vi "Derivative.vi"(10 "X":dbl[](array[numeric]), 11 "Y":dbl[](array[numeric])) -> (3 "dY/dX":dbl[](array[numeric]))   [LabVIEW 2014]
uses:
  <vilib>/Analysis/NI_AALPro.lvlib
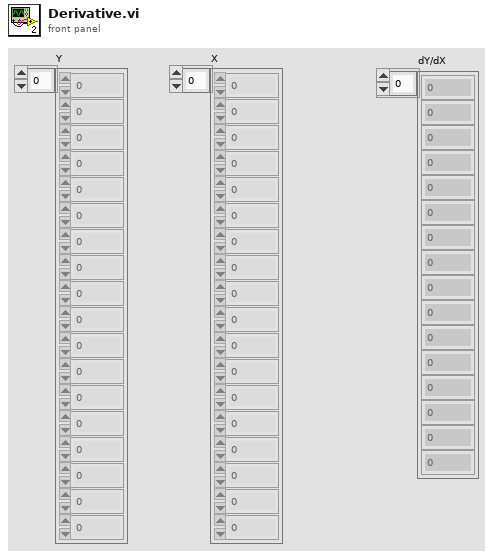
[diagram p1: front panel]
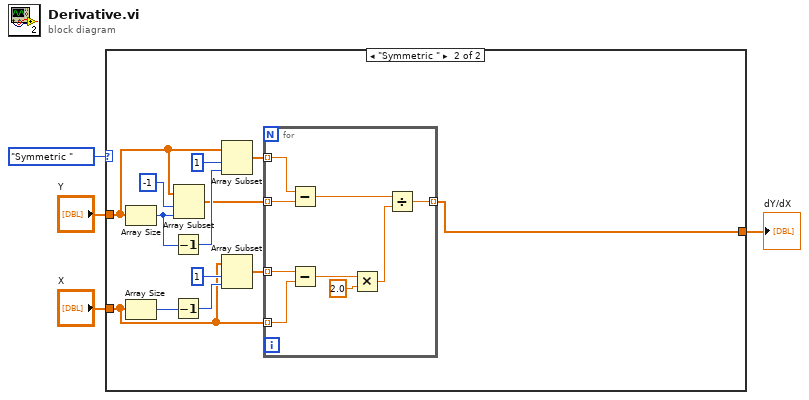
[diagram p0: block diagram]
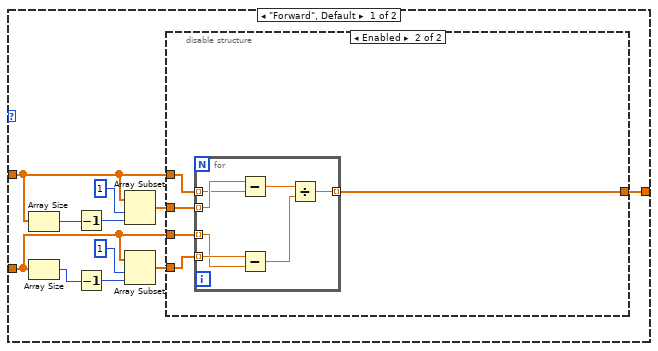
[diagram p2: hidden frame]
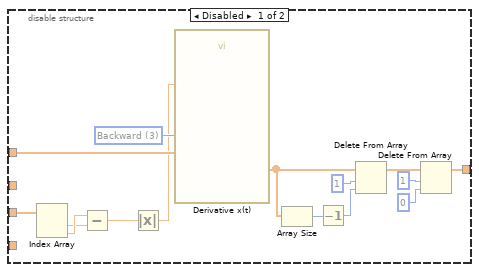
[diagram p3: hidden frame]
diagram:
  n1 = case shown="\"Symmetric \"" enum16{"Forward", "Symmetric "}."Symmetric " {
    tunnel: [w15 w43] -> w4
    tunnel: "Y" -> [w14 w48]
    tunnel: "X" -> [w6 w44]
    frame "Forward", Default {
      n2 = Array Size(array=w14) -> (size(s)=w12:i32)
      n3 = Array Size(array=w6) -> (size(s)=w9:i32)
      n4 = Decrement(x=w12) -> (x-1=w11:i32)
      n5 = Decrement(x=w9) -> (x-1=w8:i32)
      n6 = Array Subset(array=w14, index=1, length=w11) -> (w10:dbl[])
      n7 = Array Subset(array=w6, index=1, length=w8) -> (w5:dbl[])
      n8 = disable-structure shown="Enabled" {
        disable-tunnel: w14 -> [w22 w34]
        disable-tunnel: w6 -> [w21 w35]
        disable-tunnel: [w17 w31] -> w15
        disable-tunnel: w10 -> [_ w33]
        disable-tunnel: w5 -> [_ w32]
        frame Disabled {
          w30 = u16 3 items=["2nd Order Central", "4th Order Central", "Forward", "Backward"] ("method")
          n9 = Index Array(array=w21) -> (element #1=w27:dbl, element #2=w28:dbl)  [unwired: 2 in]
          n10 = Subtract(x=w28, y=w27) -> (x-y=w29:dbl)
          n11 = Absolute Value(x=w29) -> (abs(x)=w16:dbl)
          n12 = call <vilib>:"Derivative x(t).vi"("method"=w30, "dt"=w16, "X"=w22) -> ("dX/dt"=w25:dbl[])  [unwired: 7 in, 1 out]
          n13 = Array Size(array=w25) -> (size(s)=w26:i32)
          n14 = Decrement(x=w26) -> (x-1=w24:i32)
          n15 = Delete From Array(array=w25, length=1, index=w24) -> (array with subset deleted=w20:dbl[])  [unwired: 1 out]
          n16 = Delete From Array(array=w20, length=1, index=0) -> (array with subset deleted=w17:dbl[])  [unwired: 1 out]
        }
        frame Enabled {
          n17 = for {
            tunnel: w35 -> [w39] mode=indexing
            tunnel: w34 -> [w41] mode=indexing
            tunnel: w33 -> [w42] mode=indexing
            tunnel: w32 -> [w40] mode=indexing
            tunnel: [w38] -> w31 mode=indexing
            n18 = Subtract(x=w42, y=w41) -> (x-y=w37:dbl)
            n19 = Subtract(x=w40, y=w39) -> (x-y=w36:dbl)
            n20 = Divide(x=w37, y=w36) -> (x/y=w38:dbl)
          }
        }
      }
    }
    frame "Symmetric " {
      n21 = Array Size(array=w48) -> (size(s)=w49:i32)
      n22 = Array Size(array=w44) -> (size(s)=w53:i32)
      n23 = Decrement(x=w49) -> (x-1=w52:i32)
      n24 = Decrement(x=w53) -> (x-1=w55:i32)
      n25 = Array Subset(array=w48, index=-1, length=w49) -> (w46:dbl[])
      n26 = Array Subset(array=w48, index=1, length=w52) -> (w47:dbl[])
      n27 = Array Subset(array=w44, index=1, length=w55) -> (w45:dbl[])
      n28 = for {
        tunnel: w47 -> [w64] mode=indexing
        tunnel: w46 -> [w63] mode=indexing
        tunnel: w45 -> [w62] mode=indexing
        tunnel: w44 -> [w61] mode=indexing
        tunnel: [w56] -> w43 mode=indexing
        n29 = Subtract(x=w64, y=w63) -> (x-y=w58:dbl)
        n30 = Subtract(x=w62, y=w61) -> (x-y=w60:dbl)
        n31 = Multiply(x=w60, y=2.0) -> (x*y=w57:dbl)
        n32 = Divide(x=w58, y=w57) -> (x/y=w56:dbl)
      }
    }
  }
  "dY/dX" <- w4
